vi "Configure IQ Vs Slot Measurement Start Stop Index.vi"(7 "Stop Index (0)":i32, 8 "error in (no error)":errorcluster, 9 "Start Index (0)":i32, 10 "Instance (1)":i32=1, 11 "VISA resource name":refnum<visa-resource-name>) -> (0 "error out":errorcluster, 3 "VISA resource name out":refnum<visa-resource-name>)   [LabVIEW 2015, in "Rohde&Schwarz CMXP GPRF.lvlib"]
doc: "Selects the range of subsweeps to be measured (first and last subsweep of a sweep).\nThe total number of steps must not exceed 3000 (step count times number of subsweeps).\n\nAttribute:\nRSCMXPGPRF_ATTR_IQ_VS_SLOT_MEASUREMENT_START_STOP_INDEX\n\nRemote-control command:\nCONFigure:GPRF:MEAS<i>:IQVSlot:LIST:SSTop"
uses:
  <instrlib>/Rohde&Schwarz CMXP GPRF/Rohde&Schwarz CMXP GPRF.lvlib
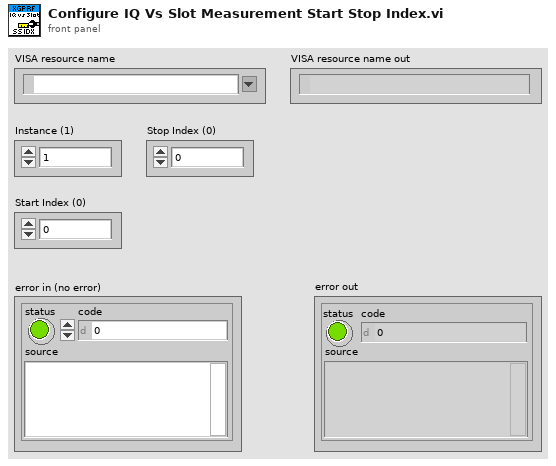
[diagram p1: front panel]
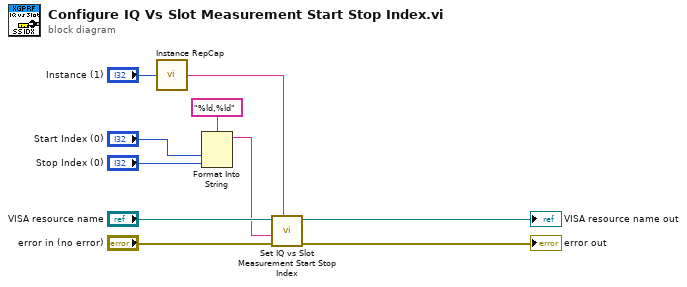
[diagram p0: block diagram]
diagram:
  n1 = call <instrlib>:"Instance RepCap.vi"("instance  in"="Instance (1)") -> ("instance out"=w5:string)
  n2 = Format Into String(format string="%ld,%ld", "Start Index (0)", "Stop Index (0)") -> (resulting string=w1:string)  [unwired: 2 in, 1 out]
  n3 = call "Set IQ vs Slot Measurement Start Stop Index"("Repeated Capabilities"=w5, "error in (no error)"="error in (no error)", "IQ vs Slot Measurement Start Stop Index ()"=w1, "instrument handle"="VISA resource name") -> ("error out"=→"error out":errorcluster, "instrument handle out"=→"VISA resource name out":refnum<visa-resource-name>)  [unwired: 6 in]
